vi "Create GPIO DAQ Task.vi"() -> ()   [LabVIEW 2018]
uses:
  <vilib>/DAQmx/create/channels.llb/DAQmx Create Channel (DO-Digital Output).vi
panel:
  in  "GPIO Ch 0":tag="DAQ_Simulator/port0/line2,DAQ_Simulator/port0/line3"
  out "concatenated string":string="PXI1Slot3/port0/line0,PXI1Slot3/port0/line3,PXI1Slot3/port0/line4,PXI1Slot3/port0/line28,PXI1Slot3/port0/line10,PXI1Slot3/port0/line4,PXI1Slot3/port0/line12,PXI1Slot3/port0/line15,PXI1Slot3/port0/line22,PXI1Slot3/port0/line23,PXI1Slot3/port0/line26,PXI1Slot3/port0/line30,PXI1Slot3/port0/line29,PXI1Slot3/port0/line19,PXI1Slot3/port0/line17,PXI1Slot3/port0/line25,PXI1Slot3/port1/line3,PXI1Slot3/port0/line24,PXI1Slot3/port1/line4"
  in  "GPIO Channels":T1={"GPIO Ch 0"="PXI1Slot3/port0/line0", "GPIO Ch 1"="PXI1Slot3/port0/line3", "GPIO Ch 2"="PXI1Slot3/port0/line4", "GPIO Ch 3"="PXI1Slot3/port0/line28", "GPIO Ch 4"="PXI1Slot3/port0/line10", "GPIO Ch 5"="PXI1Slot3/port0/line4", "GPIO Ch 6"="PXI1Slot3/port0/line12", "GPIO Ch 7"="PXI1Slot3/port0/line15", "GPIO Ch 8"="PXI1Slot3/port0/line22", "GPIO Ch 9"="PXI1Slot3/port0/line23", "GPIO Ch 10"="PXI1Slot3/port0/line26", "GPIO Ch 11"="PXI1Slot3/port0/line30", "GPIO Ch 12"="PXI1Slot3/port0/line29", "GPIO Ch 13"="PXI1Slot3/port0/line19", "GPIO Ch 14"="PXI1Slot3/port0/line17", "GPIO Ch 15"="PXI1Slot3/port0/line25", "GPIO Ch 16"="PXI1Slot3/port1/line3", "GPIO Ch 17"="PXI1Slot3/port0/line24", "GPIO Ch 18"="PXI1Slot3/port1/line4"}
  out "error out":errorcluster
  out "GPIO Task":refnum<k21>
  in  "error in":errorcluster
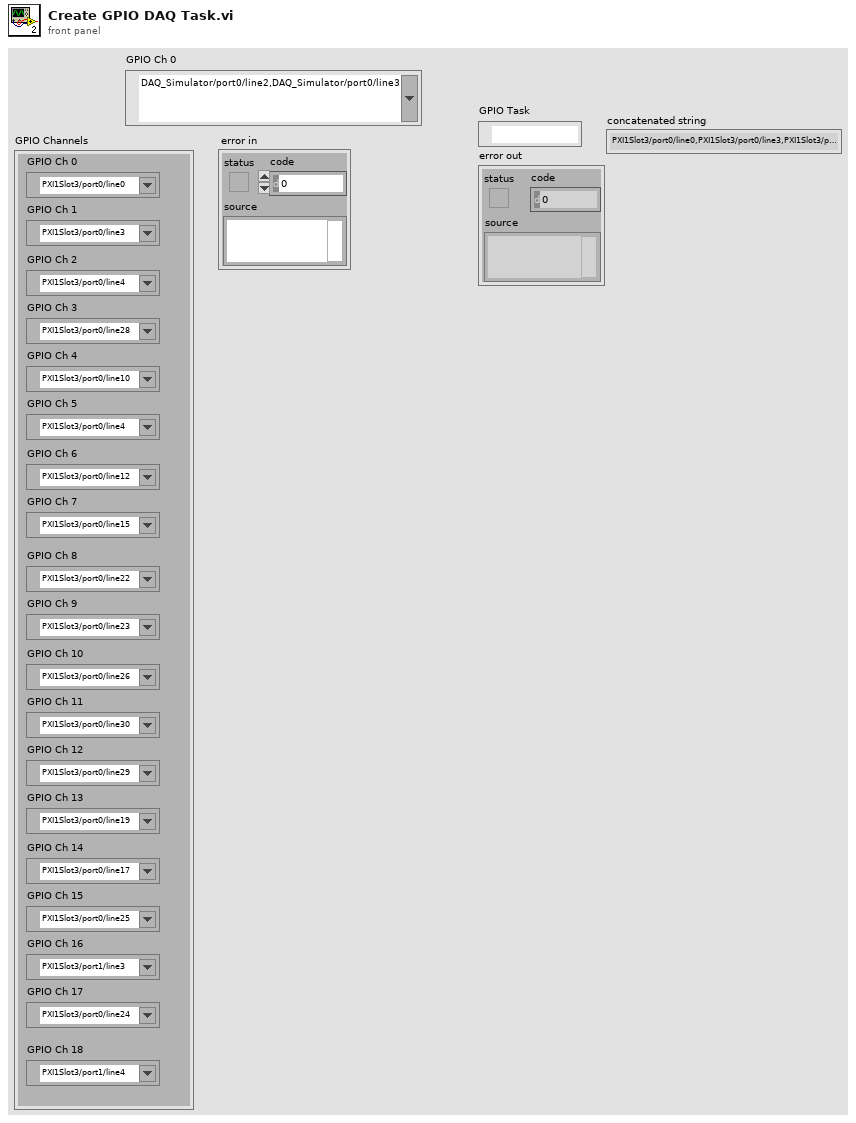
[diagram p1: front panel]
types:
  T1 = cluster{"GPIO Ch 0":tag, "GPIO Ch 1":tag, "GPIO Ch 2":tag, "GPIO Ch 3":tag, "GPIO Ch 4":tag, "GPIO Ch 5":tag, "GPIO Ch 6":tag, "GPIO Ch 7":tag, "GPIO Ch 8":tag, "GPIO Ch 9":tag, "GPIO Ch 10":tag, "GPIO Ch 11":tag, "GPIO Ch 12":tag, "GPIO Ch 13":tag, "GPIO Ch 14":tag, "GPIO Ch 15":tag, "GPIO Ch 16":tag, "GPIO Ch 17":tag, "GPIO Ch 18":tag}
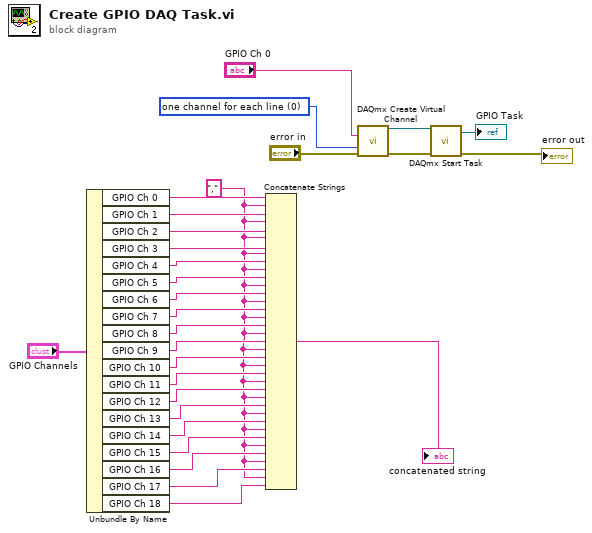
[diagram p0: block diagram]
diagram:
  w3 = "," ("string")
  w29 = 0 items=["one channel for each line", "one channel for all lines"] ("line grouping")
  n1 = Unbundle By Name("GPIO Channels") -> ("GPIO Ch 0"=w22:tag, "GPIO Ch 1"=w21:tag, "GPIO Ch 2"=w20:tag, "GPIO Ch 3"=w18:tag, "GPIO Ch 4"=w17:tag, "GPIO Ch 5"=w16:tag, "GPIO Ch 6"=w15:tag, "GPIO Ch 7"=w14:tag, "GPIO Ch 8"=w13:tag, "GPIO Ch 9"=w12:tag, "GPIO Ch 10"=w11:tag, "GPIO Ch 11"=w10:tag, "GPIO Ch 12"=w9:tag, "GPIO Ch 13"=w8:tag, "GPIO Ch 14"=w7:tag, "GPIO Ch 15"=w6:tag, "GPIO Ch 16"=w5:tag, "GPIO Ch 17"=w4:tag, "GPIO Ch 18"=w2:tag)
  n2 = Concatenate Strings(w22, w3, w21, w3, w20, w3, w18, w3, w17, w3, w16, w3, w15, w3, w14, w3, w13, w3, w12, w3, w11, w3, w10, w3, w9, w3, w8, w3, w7, w3, w6, w3, w5, w3, w4, w3, w2) -> (→"concatenated string":string)
  n3 = call-poly <vilib>:"DAQmx Create Virtual Channel.vi"("lines"="GPIO Ch 0", "line grouping"=w29, "error in"="error in") -> ("task out"=w27:refnum<k21>, "error out"=w26:errorcluster)  [unwired: 11 in]
  n4 = call <vilib>:"DAQmx Start Task.vi"("task/channels in"=w27, "error in"=w26) -> ("task out"=→"GPIO Task":refnum<k21>, "error out"=→"error out":errorcluster)  [unwired: 12 in]
